vi "Teleop.vi"(10 "Match Info":T1={"Autonomous Elapsed Seconds"=0.0, "TeleOp Elapsed Seconds"=0.0, "Disabled Elapsed Seconds"=0.0, "Visited Autonomous"=FALSE, "Visited TeleOp"=FALSE, "Visited Disabled"=FALSE, "Autonomous Settings"={"Autonomous Style"=enum."Independent", "VI Refnum"=refnum}}, 11 "Call Context":T2) -> ()   [LabVIEW 2018]
doc: "This VI is called for each TeleOp packet received from the DS where the robot is not disabled. It is often used to read from the joysticks and update I/O or to update setpoints for timed control loops. It should complete and return within 20 milliseconds or it may miss DS packets."
uses:
  <vilib>/Rock Robotics/WPI/DriverStation/WPI_DriverStationDerivedRobotMode.ctl
  <vilib>/Rock Robotics/WPI/DriverStation/WPI_DriverStationMatch Info.ctl
  <vilib>/Rock Robotics/Network Tables/NT Read Boolean.vi
  <vilib>/Rock Robotics/Network Tables/NT Read Number.vi
  <vilib>/Rock Robotics/WPI/Utilities/WPI_GetSetVariantRefNum.vi
  <vilib>/Rock Robotics/Network Tables/NT Write Boolean Array.vi
  <vilib>/Rock Robotics/Network Tables/NT Write Numeric Array.vi
  <vilib>/Rock Robotics/Network Tables/NT Read Numeric Array.vi
  <vilib>/Rock Robotics/Network Tables/NT Write Boolean.vi
  <vilib>/Rock Robotics/Network Tables/NT Write Number.vi
panel:
  in  "Motor Slow":dbl=0.75
  out "current (4)":dbl
  out "current (3)":dbl
  out "current (2)":dbl
  out "current (1)":dbl
  out "current (0)":dbl
  out "current (15)":dbl
  out "current (14)":dbl
  in  "Motor Stall":dbl format="%#_13g"
  out "Sample Slider 0":dbl(slide) scale=0.0..5.0
  out "Sample Boolean 1":bool
  out "Sample Boolean 0":bool
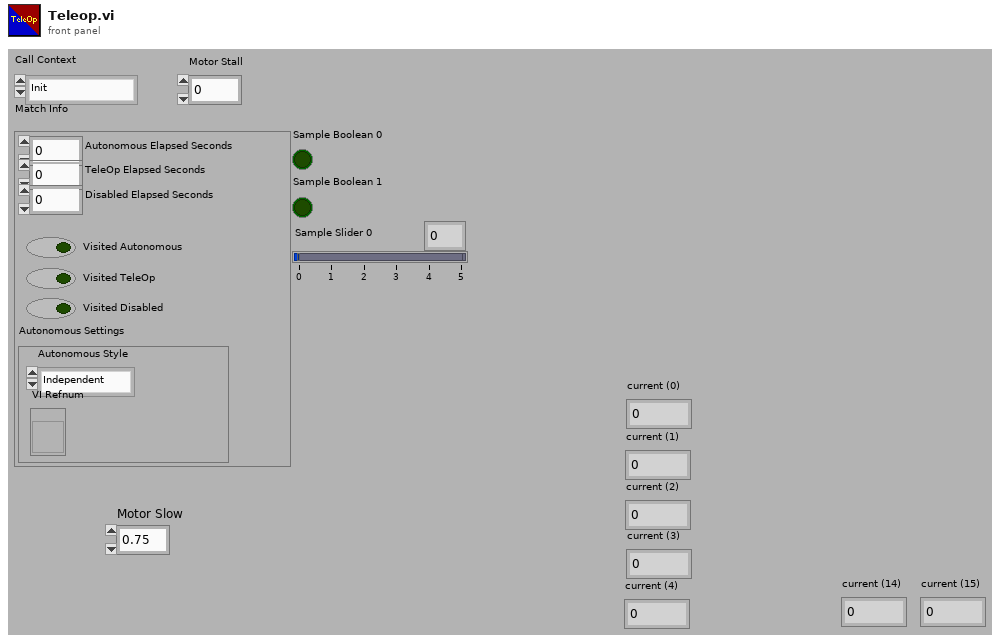
[diagram p1: front panel]
types:
  T1 = typedef "WPI_DriverStationMatch Info.ctl" = cluster{"Autonomous Elapsed Seconds":dbl, "TeleOp Elapsed Seconds":dbl, "Disabled Elapsed Seconds":dbl, "Visited Autonomous":bool, "Visited TeleOp":bool, "Visited Disabled":bool, "Autonomous Settings":cluster{"Autonomous Style":enum16{"Iterative", "Independent"}, "VI Refnum":refnum<vi>}}
  T2 = typedef "WPI_DriverStationDerivedRobotMode.ctl" = enum16{"Init", "Execute", "Stop"}
  T3 = typedef "WPI_JoystickDevRef.ctl" = cluster{"Device":T4}
  T4 = typedef "WPI_JoystickDeviceEnum.ctl" = enum16{"USB 0", "USB 1", "USB 2", "USB 3", "USB 4", "USB 5"}
  T5 = typedef "WPI_MotorControlDeviceRef.ctl" = cluster{"DeviceStatus":errorcluster, "Type":T6, "PWM":cluster{"PWM Channel":T7, "DeadBand":T8}, "CAN":cluster{"Device Number":u8, "SetOutput VI Ref":variant, "GetOutput VI Ref":variant, "Enable VI Ref":variant, "Disable VI Ref":variant, "Data":variant}, "Invert":bool, "DIO PWM":cluster{"PWM \"Enable\" Channel":T7, "DIOChannel":T9, "PWM Rate":dbl}}
  T6 = typedef "WPI_MotorControlType.ctl" = enum16{"PWM", "CAN", "DIO PWM"}
  T7 = typedef "FPGA_DIOPWMChannel.ctl" = enum8{"PWM 0", "PWM 1", "PWM 2", "PWM 3", "PWM 4", "PWM 5", "PWM 6", "PWM 7", "PWM 8", "PWM 9", "PWM MXP 0", "PWM MXP 1", "PWM MXP 2", "PWM MXP 3", "PWM MXP 4", "PWM MXP 5", "PWM MXP 6", "PWM MXP 7", "PWM MXP 8", "PWM MXP 9", "Invalid"}
  T8 = typedef "WPI_PWMDeadband.ctl" = cluster{"Name":string, "maxPositivePwm":i32, "minPositivePwm":i32, "centerPwm":i32, "maxNegativePwm":i32, "minNegativePwm":i32, "angularRange":u16}
  T9 = typedef "FPGA_DIOChannel.ctl" = enum8{"DIO 0", "DIO 1", "DIO 2", "DIO 3", "DIO 4", "DIO 5", "DIO 6", "DIO 7", "DIO 8", "DIO 9", "DIO MXP 0", "DIO MXP 1", "DIO MXP 2", "DIO MXP 3", "DIO MXP 4", "DIO MXP 5", "DIO MXP 6", "DIO MXP 7", "DIO MXP 8", "DIO MXP 9", "DIO MXP 10", "DIO MXP 11", "DIO MXP 12", "DIO MXP 13", "DIO MXP 14", "DIO MXP 15", "SPI Port CS1", "SPI Port CS2", "SPI Port CS3", "SPI Port MISO", "SPI Port MOSI", "Invalid"}
  T10 = typedef "WPI_RobotDriveDevRef.ctl" = cluster{"DevStatus":errorcluster, "Motors[]":T5[], "Square Inputs":bool, "Max Output":dbl}
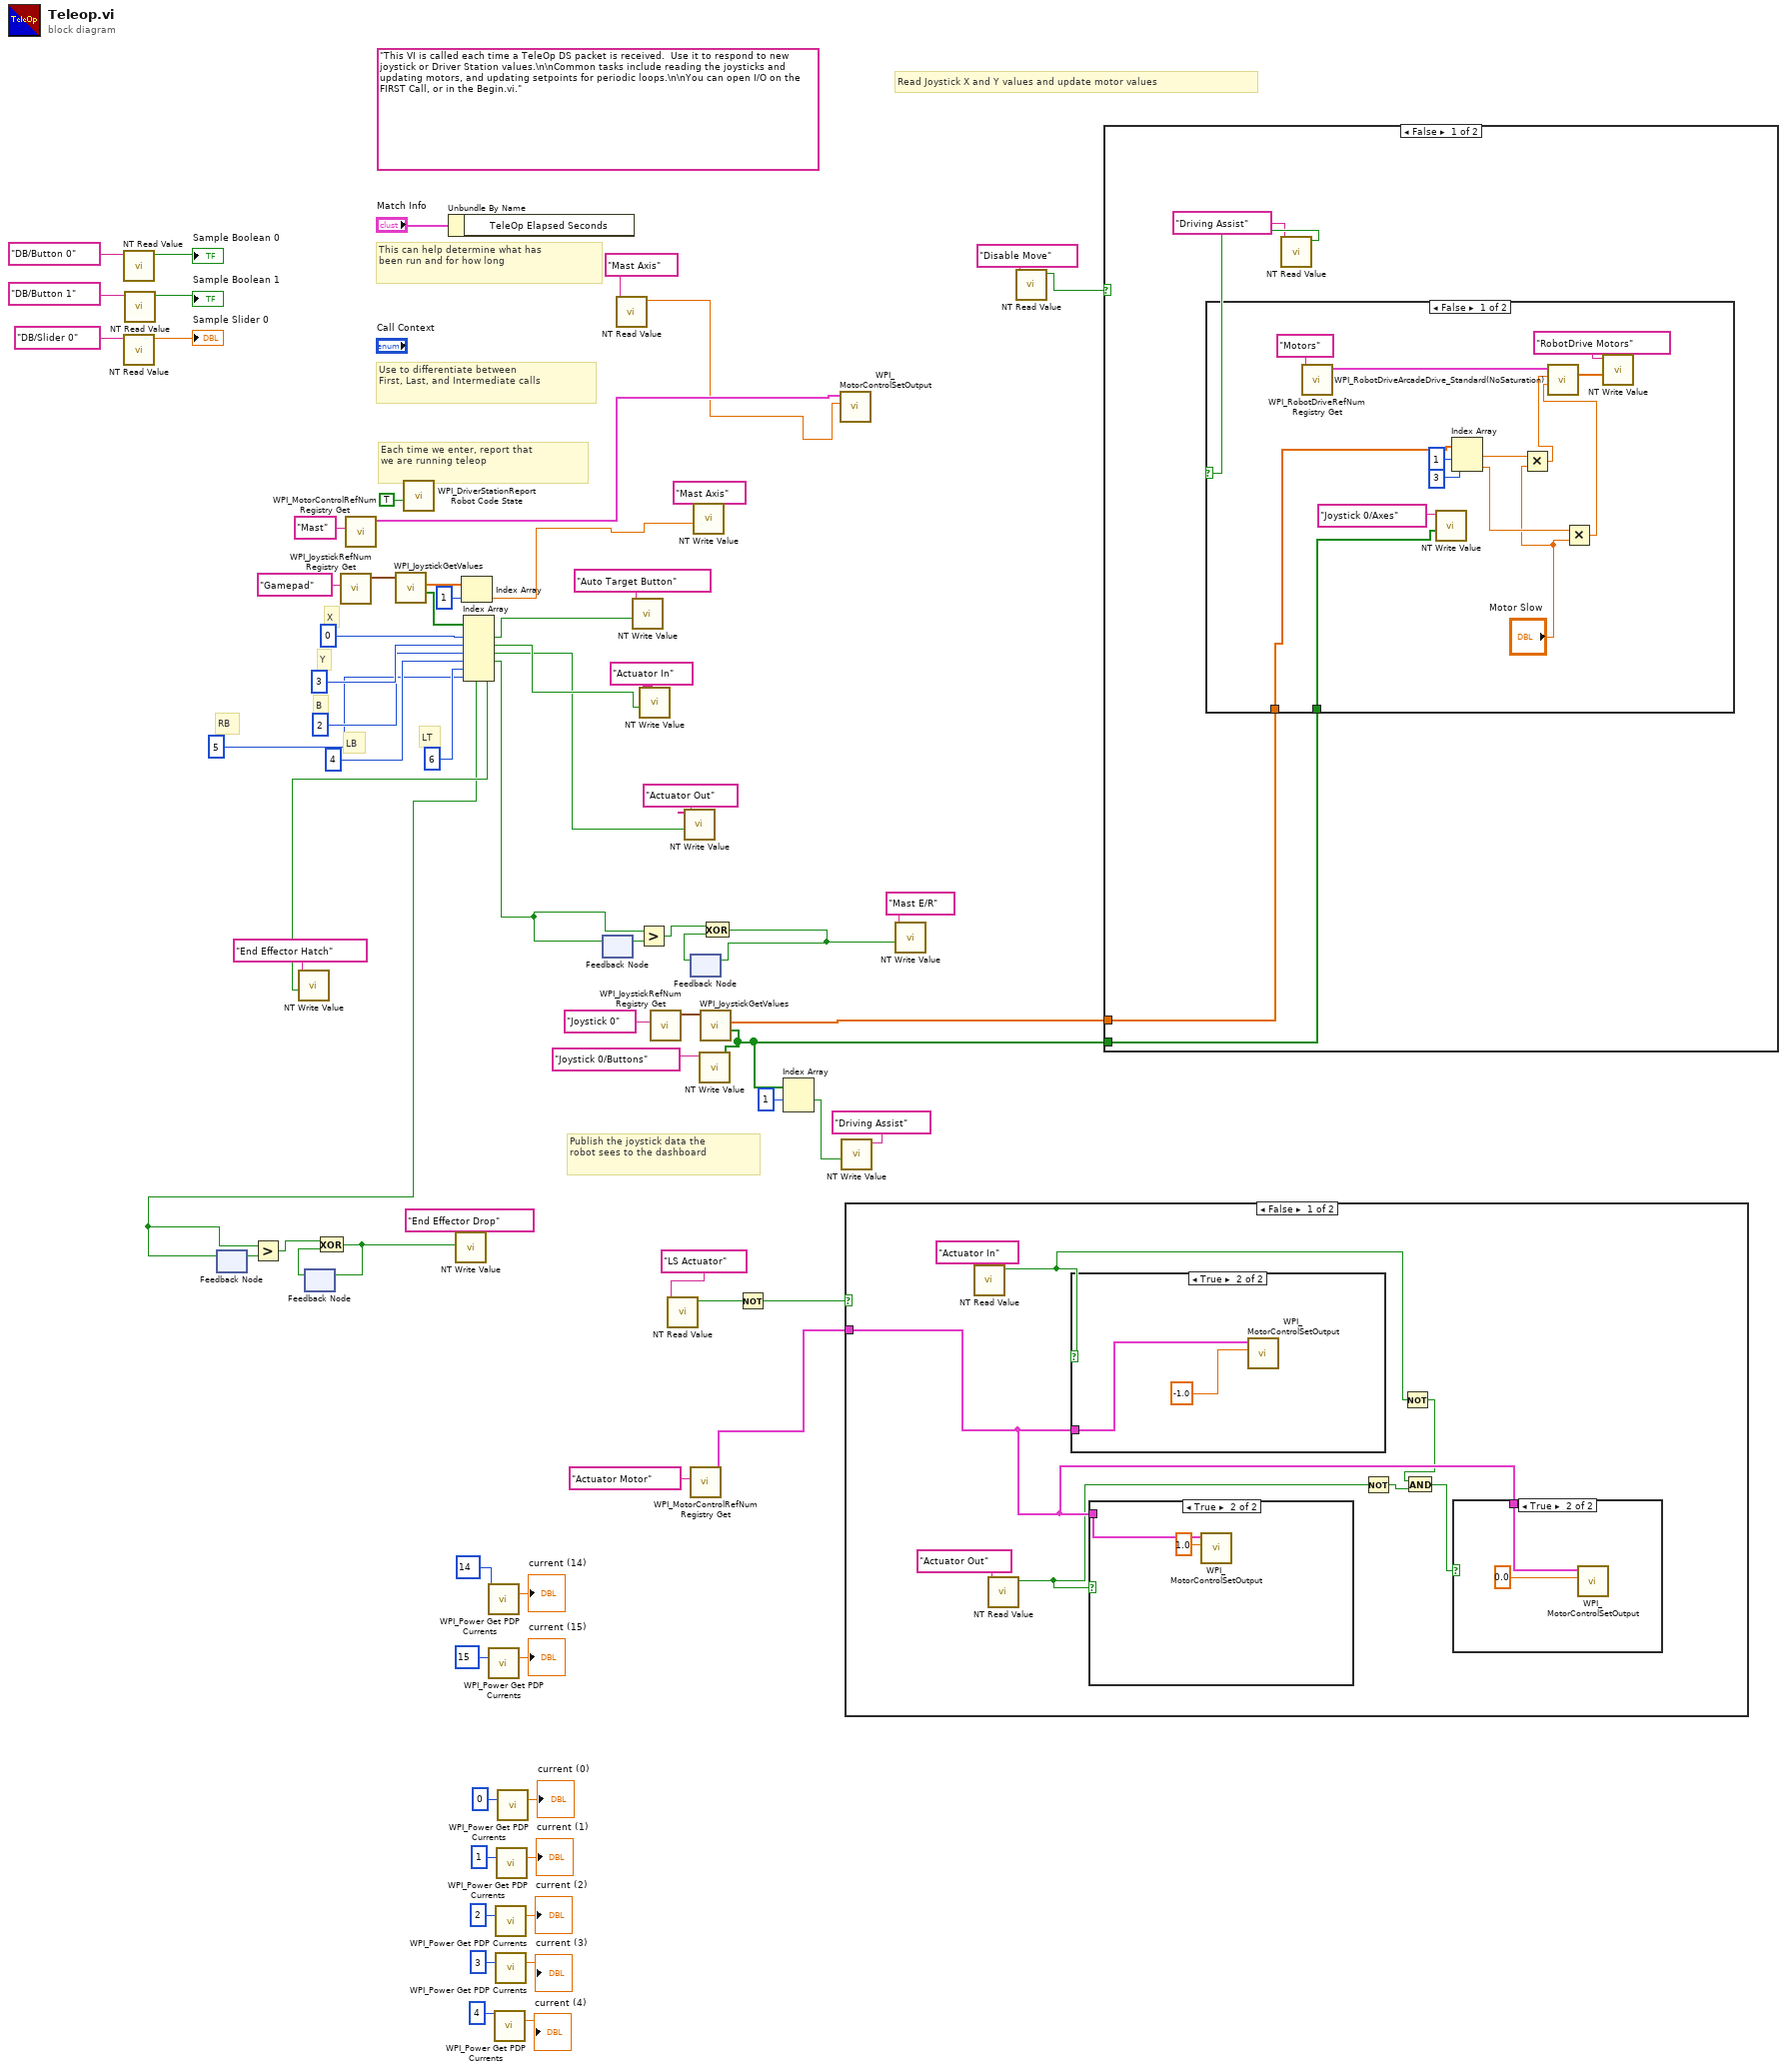
[diagram p0: block diagram]
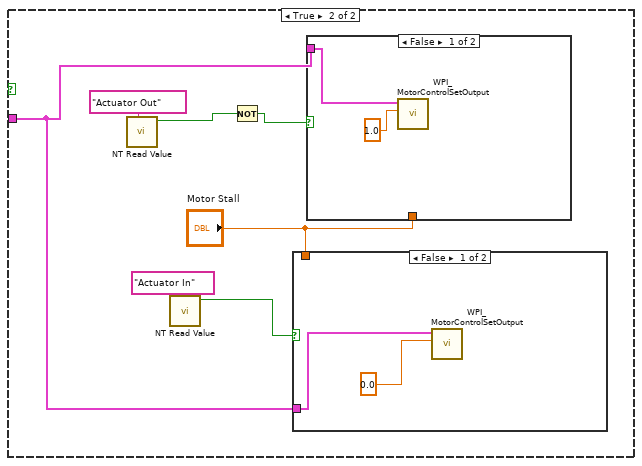
[diagram p5: hidden frame]
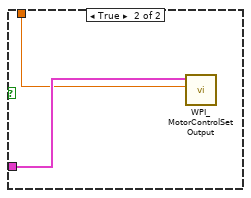
[diagram p6: hidden frame]
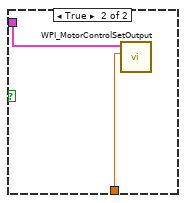
[diagram p7: hidden frame]
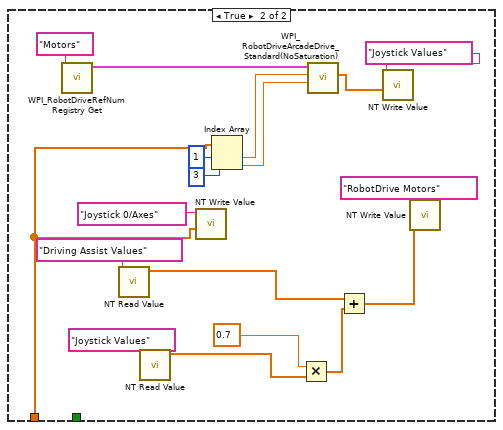
[diagram p8: hidden frame]
diagram:
  (unwired) "This VI is called each time a TeleOp DS packet is received.  Use it to respond to new joystick or Driver Station values.\n\nCommon tasks include reading the joysticks and updating motors, and updating setpoints for periodic loops.\n\nYou can open I/O on the FIRST Call, or in the Begin.vi."
  # "RB"
  # "LT"
  # "LB"
  # "Publish the joystick data the\nrobot sees to the dashboard"
  # "B"
  # "X"
  # "Y"
  # "Each time we enter, report that\nwe are running teleop"
  # "Use to differentiate between\nFirst, Last, and Intermediate calls"
  # "This can help determine what has\nbeen run and for how long"
  # "Read Joystick X and Y values and update motor values"
  n1 = call-poly <vilib>:"NT Read Value.vi"("Name"="DB/Button 0" ("refnum name")) -> ("Boolean"=→"Sample Boolean 0":bool)  [unwired: 9 in, 1 out]
  n2 = call-poly <vilib>:"NT Read Value.vi"("Name"="DB/Slider 0" ("refnum name")) -> ("Numeric"=→"Sample Slider 0":dbl)  [unwired: 9 in, 1 out]
  n3 = call-poly <vilib>:"NT Read Value.vi"("Name"="DB/Button 1" ("refnum name")) -> ("Boolean"=→"Sample Boolean 1":bool)  [unwired: 9 in, 1 out]
  n4 = feedback #1() -> (w20:bool)  [unwired: 1 in]
  n5 = feedback #2() -> (w18:bool)  [unwired: 1 in]
  n6 = call <vilib>:"WPI_JoystickRefNum Registry Get.vi"("refnum name"="Gamepad") -> ("JoystickDevRef"=w64:T3)  [unwired: 9 in, 1 out]
  n7 = call <vilib>:"WPI_MotorControlRefNum Registry Get.vi"("refnum name"="Mast") -> ("MotorControlDevRef"=w27:T5)  [unwired: 9 in, 1 out]
  n8 = call <vilib>:"WPI_JoystickGetValues.vi"("JoystickDevRef"=w64) -> ("Buttons"=w59:bool[], "Axes"=w63:dbl[])  [unwired: 6 in, 3 out]
  n9 = call <vilib>:"WPI_DriverStationReport Robot Code State.vi"("TeleOp"=TRUE ("Autonomous")) -> ()  [unwired: 10 in, 1 out]
  n10 = Unbundle By Name("Match Info") -> ()  [unwired: 1 out]
  n11 = Index Array(array=w63, index=1) -> (element=w30:dbl)
  n12 = Index Array(array=w59, index #1=0 ("index"), index #2=3 ("index"), index #3=2 ("index"), index #4=4 ("index"), index #5=6 ("index"), index #6=5 ("index")) -> (element #1=w57:bool, element #2=w51:bool, element #3=w48:bool, element #4=w25:bool, element #5=w17:bool, element #6=w35:bool)
  n13 = feedback-in #1(w17) -> ()
  n14 = Greater?(x=w17, y=w20) -> (0:w19:bool)
  n15 = call-poly <vilib>:"NT Write Value.vi"("Boolean"=w35, "Name"="End Effector Hatch") -> ()  [unwired: 9 in, 1 out]
  n16 = Exclusive Or(1:w18, 2:w19) -> (0:w16:bool)
  n17 = feedback-in #2(w16) -> ()
  n18 = call-poly <vilib>:"NT Write Value.vi"("Boolean"=w16, "Name"="End Effector Drop") -> ()  [unwired: 9 in, 1 out]
  n19 = call <vilib>:"WPI_Power Get PDP Currents.vi"("PDP Channel"=14) -> ("current (A)"=→"current (14)":dbl)  [unwired: 12 in, 2 out]
  n20 = call <vilib>:"WPI_Power Get PDP Currents.vi"("PDP Channel"=15) -> ("current (A)"=→"current (15)":dbl)  [unwired: 12 in, 2 out]
  n21 = call <vilib>:"WPI_Power Get PDP Currents.vi"("Power Distribution Panel (0)"=u8 4) -> ("current (A)"=→"current (4)":dbl)  [unwired: 12 in, 2 out]
  n22 = call <vilib>:"WPI_Power Get PDP Currents.vi"("PDP Channel"=2) -> ("current (A)"=→"current (2)":dbl)  [unwired: 12 in, 2 out]
  n23 = call <vilib>:"WPI_Power Get PDP Currents.vi"("PDP Channel"=3) -> ("current (A)"=→"current (3)":dbl)  [unwired: 12 in, 2 out]
  n24 = call <vilib>:"WPI_Power Get PDP Currents.vi"("PDP Channel"=1) -> ("current (A)"=→"current (1)":dbl)  [unwired: 12 in, 2 out]
  n25 = call <vilib>:"WPI_Power Get PDP Currents.vi"("PDP Channel"=0) -> ("current (A)"=→"current (0)":dbl)  [unwired: 12 in, 2 out]
  n26 = feedback #3() -> (w24:bool)  [unwired: 1 in]
  n27 = feedback-in #3(w25) -> ()
  n28 = call-poly <vilib>:"NT Read Value.vi"("Name"="Mast Axis") -> ("Numeric"=w26:dbl)  [unwired: 9 in, 1 out]
  n29 = call-poly <vilib>:"NT Write Value.vi"("Boolean"=w57, "Name"="Auto Target Button") -> ()  [unwired: 9 in, 1 out]
  n30 = Greater?(x=w25, y=w24) -> (0:w23:bool)
  n31 = call-poly <vilib>:"NT Write Value.vi"("Boolean"=w51, "Name"="Actuator In") -> ()  [unwired: 9 in, 1 out]
  n32 = call <vilib>:"WPI_JoystickRefNum Registry Get.vi"("refnum name"="Joystick 0") -> ("JoystickDevRef"=w45:T3)  [unwired: 1 in, 9 out]
  n33 = call-poly <vilib>:"NT Read Value.vi"("Name"="LS Actuator") -> ("Boolean"=w54:bool)  [unwired: 9 in, 1 out]
  n34 = call-poly <vilib>:"NT Write Value.vi"("Boolean"=w48, "Name"="Actuator Out") -> ()  [unwired: 9 in, 1 out]
  n35 = feedback #4() -> (w21:bool)  [unwired: 1 in]
  n36 = call <vilib>:"WPI_MotorControlRefNum Registry Get.vi"("refnum name"="Actuator Motor") -> ("MotorControlDevRef"=w46:T5)  [unwired: 9 in, 1 out]
  n37 = call-poly <vilib>:"NT Write Value.vi"("Numeric"=w30, "Name"="Mast Axis") -> ()  [unwired: 9 in, 1 out]
  n38 = call <vilib>:"WPI_JoystickGetValues.vi"("JoystickDevRef"=w45) -> ("Buttons"=w41:bool[], "Axes"=w43:dbl[])  [unwired: 6 in, 3 out]
  n39 = call-poly <vilib>:"NT Write Value.vi"("Boolean Array"=w41, "Name"="Joystick 0/Buttons") -> ()  [unwired: 9 in, 1 out]
  n40 = Exclusive Or(1:w21, 2:w23) -> (0:w22:bool)
  n41 = feedback-in #4(w22) -> ()
  n42 = Not(x=w54) -> (.not. x?=w1:bool)
  n43 = Index Array(array=w41, index #1=1 ("index")) -> (element #1=w39:bool)  [unwired: 1 in, 1 out]
  n44 = call <vilib>:"WPI_MotorControlSetOutput.vi"("Output"=w26, "MotorControlDevRef"=w27) -> ()  [unwired: 7 in, 3 out]
  n45 = call-poly <vilib>:"NT Write Value.vi"("Boolean"=w39, "Name"="Driving Assist") -> ()  [unwired: 9 in, 1 out]
  n46 = case shown="False" w1 {
    tunnel: w46 -> [w79 w90]
    frame False {
      n47 = call-poly <vilib>:"NT Read Value.vi"("Name"="Actuator In") -> ("Boolean"=w76:bool)  [unwired: 9 in, 1 out]
      n48 = call-poly <vilib>:"NT Read Value.vi"("Name"="Actuator Out") -> ("Boolean"=w77:bool)  [unwired: 9 in, 1 out]
      n49 = case shown="True" w76 {
        tunnel: w79 -> [_ w87]
        frame False {
        }
        frame True {
          n50 = call <vilib>:"WPI_MotorControlSetOutput.vi"("Output"=-1.0, "MotorControlDevRef"=w87) -> ()  [unwired: 7 in, 3 out]
        }
      }
      n51 = case shown="True" w77 {
        tunnel: w79 -> [_ w86]
        frame False {
        }
        frame True {
          n52 = call <vilib>:"WPI_MotorControlSetOutput.vi"("Output"=1.0, "MotorControlDevRef"=w86) -> ()  [unwired: 7 in, 3 out]
        }
      }
      n53 = Not(x=w77) -> (.not. x?=w78:bool)
      n54 = Not(x=w76) -> (.not. x?=w75:bool)
      n55 = And(x=w75, y=w78) -> (x .and. y?=w80:bool)
      n56 = case shown="True" w80 {
        tunnel: w79 -> [_ w83]
        frame False {
        }
        frame True {
          n57 = call <vilib>:"WPI_MotorControlSetOutput.vi"("Output"=0.0, "MotorControlDevRef"=w83) -> ()  [unwired: 7 in, 3 out]
        }
      }
    }
    frame True {
      n58 = call-poly <vilib>:"NT Read Value.vi"("Name"="Actuator Out") -> ("Boolean"=w94:bool)  [unwired: 9 in, 1 out]
      n59 = call-poly <vilib>:"NT Read Value.vi"("Name"="Actuator In") -> ("Boolean"=w91:bool)  [unwired: 9 in, 1 out]
      n60 = Not(x=w94) -> (.not. x?=w93:bool)
      n61 = case shown="False" w91 {
        tunnel: w90 -> [w96 w99]
        tunnel: "Motor Stall" -> [_ w98]
        frame False {
          n62 = call <vilib>:"WPI_MotorControlSetOutput.vi"("Output"=0.0, "MotorControlDevRef"=w96) -> ()  [unwired: 7 in, 3 out]
        }
        frame True {
          n63 = call <vilib>:"WPI_MotorControlSetOutput.vi"("Output"=w98, "MotorControlDevRef"=w99) -> ()  [unwired: 7 in, 3 out]
        }
      }
      n64 = case shown="False" w93 {
        tunnel: w90 -> [w101 w103]
        tunnel: "Motor Stall" -> [_ w102]
        frame False {
          n65 = call <vilib>:"WPI_MotorControlSetOutput.vi"("Output"=1.0, "MotorControlDevRef"=w101) -> ()  [unwired: 7 in, 3 out]
        }
        frame True {
          n66 = call <vilib>:"WPI_MotorControlSetOutput.vi"("Output"=w102, "MotorControlDevRef"=w103) -> ()  [unwired: 7 in, 3 out]
        }
      }
    }
  }
  n67 = call-poly <vilib>:"NT Write Value.vi"("Boolean"=w22, "Name"="Mast E/R") -> ()  [unwired: 9 in, 1 out]
  n68 = call-poly <vilib>:"NT Read Value.vi"("Name"="Disable Move") -> ("Boolean"=w61:bool)  [unwired: 9 in, 1 out]
  n69 = case shown="False" w61 {
    tunnel: w41 -> [w106 _]
    tunnel: w43 -> [w107 _]
    frame False {
      n70 = call-poly <vilib>:"NT Read Value.vi"("Name"="Driving Assist") -> ("Boolean"=w105:bool)  [unwired: 9 in, 1 out]
      n71 = case shown="False" w105 {
        tunnel: w107 -> [w114 w132]
        tunnel: w106 -> [w113 _]
        frame False {
          n72 = call <vilib>:"WPI_RobotDriveRefNum Registry Get.vi"("refnum name"="Motors") -> ("RobotDriveDevRef"=w120:T10)  [unwired: 1 in, 9 out]
          n73 = call-poly <vilib>:"NT Write Value.vi"("Boolean Array"=w113, "Name"="Joystick 0/Axes") -> ()  [unwired: 9 in, 1 out]
          n74 = Index Array(array=w114, index #1=1 ("index"), index #2=3 ("index")) -> (element #1=w109:dbl, element #2=w112:dbl)
          n75 = Multiply(x=w109, y="Motor Slow") -> (x*y=w108:dbl)
          n76 = Multiply(x=w112, y="Motor Slow") -> (x*y=w111:dbl)
          n77 = call <vilib>:"WPI_RobotDriveArcadeDrive_Standard(NoSaturation).vi"("Y axis value"=w111, "X axis value"=w108, "RobotDriveDevRef"=w120) -> ("Motor Values"=w118:dbl[])  [unwired: 1 in, 7 out]
          n78 = call-poly <vilib>:"NT Write Value.vi"("Numeric Array"=w118, "Name"="RobotDrive Motors") -> ()  [unwired: 9 in, 1 out]
        }
        frame True {
          n79 = call <vilib>:"WPI_RobotDriveRefNum Registry Get.vi"("refnum name"="Motors") -> ("RobotDriveDevRef"=w138:T10)  [unwired: 1 in, 9 out]
          n80 = call-poly <vilib>:"NT Read Value.vi"("Name"="Driving Assist Values") -> ("Numeric Array"=w127:dbl[])  [unwired: 9 in, 1 out]
          n81 = call-poly <vilib>:"NT Read Value.vi"("Name"="Joystick Values") -> ("Numeric Array"=w125:dbl[])  [unwired: 9 in, 1 out]
          n82 = call-poly <vilib>:"NT Write Value.vi"("Numeric Array"=w132, "Name"="Joystick 0/Axes") -> ()  [unwired: 9 in, 1 out]
          n83 = Index Array(array=w132, index #1=1 ("index"), index #2=3 ("index")) -> (element #1=w137:dbl, element #2=w136:dbl)
          n84 = Multiply(x=0.7, y=w125) -> (x*y=w122:dbl[])
          n85 = call <vilib>:"WPI_RobotDriveArcadeDrive_Standard(NoSaturation).vi"("Y axis value"=w136, "X axis value"=w137, "RobotDriveDevRef"=w138) -> ("Motor Values"=w130:dbl[])  [unwired: 1 in, 7 out]
          n86 = Add(x=w127, y=w122) -> (x+y=w123:dbl[])
          n87 = call-poly <vilib>:"NT Write Value.vi"("Numeric Array"=w130, "Name"="Joystick Values") -> ()  [unwired: 9 in, 1 out]
          n88 = call-poly <vilib>:"NT Write Value.vi"("Numeric Array"=w123, "Name"="RobotDrive Motors") -> ()  [unwired: 9 in, 1 out]
        }
      }
    }
    frame True {
    }
  }
